vi "NML VISA Open Conditional.vi"(8 "error in (no error)":errorcluster {"code" format="%.0x"}, 11 "VISA resource name":refnum<visa-resource-name>) -> (0 "error out":errorcluster {"code" format="%.0x"}, 2 "Opened?":bool, 3 "dup VISA Session":refnum<visa-resource-name>)   [LabVIEW 2020]
uses:
  Sub Controls/VISA Session Status.ctl
  <vilib>/regexp/Match Regular Expression.xnode
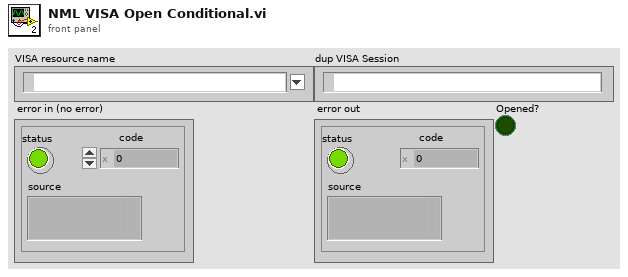
[diagram p1: front panel]
types:
  T1 = typedef "VISA Session Status.ctl" = enum16{"VISA Session Closed", "VISA Session Open", "VISA Session Locked"}
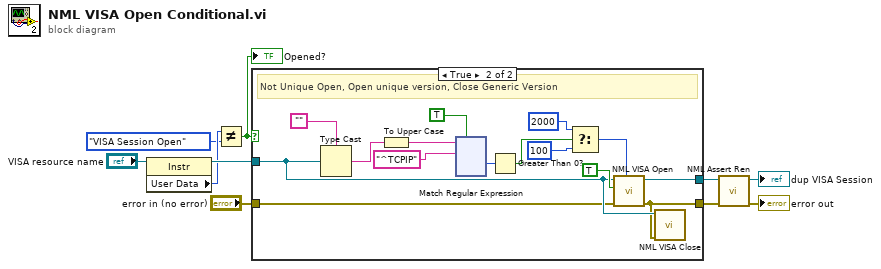
[diagram p0: block diagram]
diagram:
  n1 = property class="Instr"(reference="VISA resource name") -> (reference out=w4:refnum<visa-resource-name>, "User Data"=w3:u32)  [unwired: 1 in, 1 out]
  n2 = Not Equal?(x=w3, y=VISA_Session_Status."VISA Session Open") -> (x != y?=w2:bool)
  "Opened?" <- w2
  n3 = case shown="True" w2 {
    tunnel: w4 -> [w12 w15]
    tunnel: "error in (no error)" -> [w11 w14]
    tunnel: [w12 w27] -> w7
    tunnel: [w11 w13] -> w6
    frame False {
      # "Already Opened by NML Open Function"
    }
    frame True {
      # "Not Unique Open, Open unique version, Close Generic Version"
      n4 = Type Cast(type="", x=w15) -> (*(type *) &x=w20:string)
      n5 = To Upper Case(1:w20) -> (0:w16:string)
      n6 = xnode "Match Regular Expression"("input string"=w16, "regular expression"="^TCPIP", "ignore case? (F)"=TRUE) -> ("offset past match"=w18:i32)  [unwired: 3 in, 4 out]
      n7 = Greater Than 0?(x=w18) -> (x > 0?=w17:bool)
      n8 = Select(t=u32 2000 ("VISA Open timeout (0)"), s=w17, f=u32 100) -> (s? t:f=w23:u32)
      n9 = call "NML VISA Open.vi"("VISA Open timeout (0)"=w23, "error in (no error)"=w14, "duplicate session (T)"=TRUE, "VISA resource name"=w15) -> ("error out"=w13:errorcluster, "VISA resource name out"=w27:refnum<visa-resource-name>)  [unwired: 6 in]
      n10 = call "NML VISA Close.vi"("Error In"=w13, "VISA resource name"=w15) -> ()  [unwired: 9 in, 1 out]
    }
  }
  n11 = call "NML Assert Ren.vi"("error in (no error)"=w6, "VISA resource name"=w7) -> ("error out"=→"error out":errorcluster, "dup VISA Session"=→"dup VISA Session":refnum<visa-resource-name>)  [unwired: 8 in]
